vi "Motion FIFO.vi"(9 "Packet Length":i32, 10 "Data":i32[](array[numeric]), 11 "Motion FIFO":refnum<queue>) -> (2 "Number of Packets":i32, 3 "Array":i32[](array[numeric]))   [LabVIEW 2014]
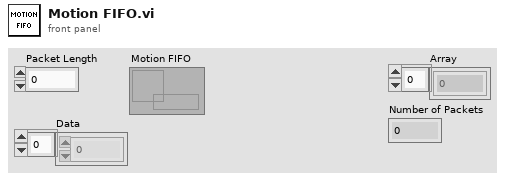
[diagram p1: front panel]
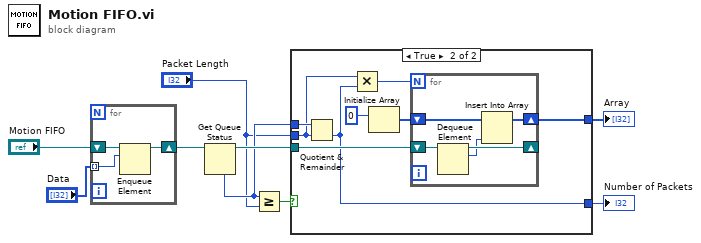
[diagram p0: block diagram]
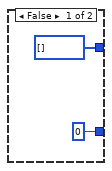
[diagram p2: hidden frame]
diagram:
  n1 = for {
    tunnel: "Data" -> [w12] mode=indexing
    shift-right: [w10] -> w7
    shift-left: "Motion FIFO" -> [w11]
    n2 = Enqueue Element(queue=w11, element=w12) -> (queue out=w10:refnum<queue>)  [unwired: 2 in, 2 out]
  }
  n3 = Get Queue Status(queue=w7) -> (queue out=w5:refnum<queue>, # elements in queue=w3:i32)  [unwired: 2 in, 6 out]
  n4 = Greater Or Equal?(x=w3, y="Packet Length") -> (x >= y?=w6:bool)
  n5 = case shown="True" w6 {
    tunnel: w5 -> [_ w22]
    tunnel: [i32[] [] w20] -> w4
    tunnel: w3 -> [_ w18]
    tunnel: "Packet Length" -> [_ w15]
    tunnel: [0 w16] -> w1
    frame False {
    }
    frame True {
      n6 = Quotient & Remainder(x=w18, y=w15) -> (floor(x/y)=w16:i32)  [unwired: 1 out]
      n7 = Multiply(x=w15, y=w16) -> (x*y=w17:i32)
      n8 = Initialize Array(0 ("element")) -> (w21:i32[])  [unwired: 1 in]
      n9 = for {
        N: w17 -> [_]
        shift-right: [w26] -> _
        shift-left: w22 -> [w27]
        shift-right: [w23] -> w20
        shift-left: w21 -> [w24]
        n10 = Dequeue Element(queue=w27) -> (queue out=w26:refnum<queue>, element=w25:i32)  [unwired: 2 in, 2 out]
        n11 = Insert Into Array(array=w24, new element=w25) -> (w23:i32[])  [unwired: 1 in]
      }
    }
  }
  "Array" <- w4
  "Number of Packets" <- w1
